vi "getProcessName.vi"(10 "Lotno":string) -> (2 "ProcessName":string)   [LabVIEW 2012]
uses:
  <vilib>/addons/database/Auxilliary.llb/DB Tools Cursor Type.ctl
  <vilib>/addons/database/Connection.llb/DB Tools Open Connec (Path).vi
  <vilib>/addons/database/Connection.llb/Conn Execute.vi
  <vilib>/addons/database/Recordset.llb/Rec Fetch Integer Data (R).vi
  <vilib>/addons/database/Recordset.llb/Rec Destroy - Connection.vi
  <vilib>/addons/database/Recordset.llb/Rec Fetch Recordset Data (R).vi
  <vilib>/addons/database/_DB Variant To Data/Database Variant To Data.xnode
  <vilib>/addons/database/NI_Database_API.lvlib
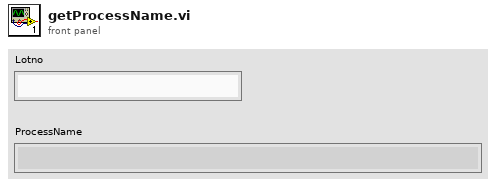
[diagram p1: front panel]
types:
  T1 = typedef "NI_Database_API.lvlib/DB Tools Cursor Type.ctl" = enum16{"forward-only", "keyset", "dynamic", "static"}
  T2 = typedef "NI_Database_API.lvlib/Conn ObjectReference.ctl" = refnum<k1>
  T3 = typedef "NI_Database_API.lvlib/Rec ObjectReference.ctl" = refnum<k1>
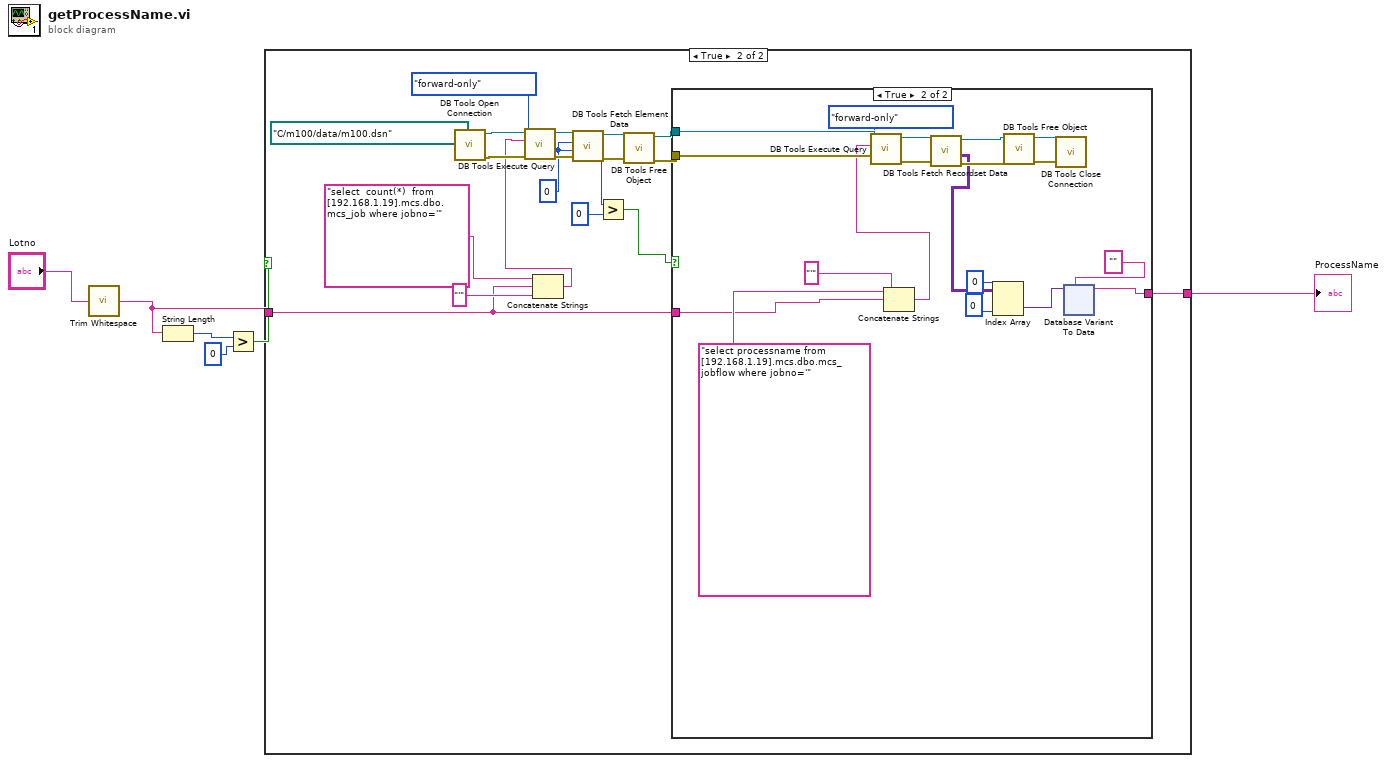
[diagram p0: block diagram]
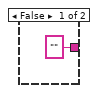
[diagram p2: hidden frame]
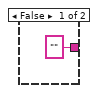
[diagram p3: hidden frame]
diagram:
  n1 = call <vilib>:"Trim Whitespace.vi"("string"="Lotno") -> ("trimmed string"=w2:string)  [unwired: 1 in]
  n2 = String Length(string=w2) -> (length=w6:i32)
  n3 = Greater?(x=w6, y=0) -> (0:w4:bool)
  n4 = case shown="True" w4 {
    tunnel: w2 -> [_ w19]
    tunnel: ["" ("data") w26] -> w1
    frame False {
    }
    frame True {
      w12 = 0
      n5 = call-poly <vilib>:"DB Tools Open Connection.vi"("connection information"=path "C:/m100/data/m100.dsn") -> ("error out"=w22:errorcluster, "connection reference"=w23:T2)  [unwired: 7 in]
      n6 = Concatenate Strings("select  count(*)  from [192.168.1.19].mcs.dbo.mcs_job where jobno='" ("string"), w19, "'" ("string")) -> (w17:string)
      n7 = call-poly <vilib>:"DB Tools Execute Query.vi"("error in (no error)"=w22, "cursor type"=DB_Tools_Cursor_Type."forward-only", "SQL query"=w17, "connection reference"=w23) -> ("error out"=w16:errorcluster, "recordset reference"=w15:T3)  [unwired: 4 in]
      n8 = call-poly <vilib>:"DB Tools Fetch Element Data.vi"("error in (no error)"=w16, "type"=w12, "column index"=w12, "recordset reference"=w15) -> ("error out"=w13:errorcluster, "data"=w11:i32, "recordset reference out"=w14:T3)  [unwired: 3 in]
      n9 = Greater?(x=w11, y=0) -> (0:w9:bool)
      n10 = call-poly <vilib>:"DB Tools Free Object.vi"("error in (no error)"=w13, "recordset reference"=w14) -> ("error out"=w24:errorcluster, "connection reference"=w25:T2)  [unwired: 8 in]
      n11 = case shown="True" w9 {
        tunnel: w25 -> [_ w44]
        tunnel: w24 -> [_ w41]
        tunnel: w19 -> [_ w32]
        tunnel: ["" ("data") w31] -> w26
        frame False {
        }
        frame True {
          n12 = Concatenate Strings("select processname from [192.168.1.19].mcs.dbo.mcs_jobflow where jobno='" ("string"), w32, "'" ("string")) -> (w35:string)
          n13 = call-poly <vilib>:"DB Tools Execute Query.vi"("error in (no error)"=w41, "cursor type"=DB_Tools_Cursor_Type."forward-only", "SQL query"=w35, "connection reference"=w44) -> ("error out"=w40:errorcluster, "recordset reference"=w43:T3)  [unwired: 4 in]
          n14 = call-poly <vilib>:"DB Tools Fetch Recordset Data.vi"("error in (no error)"=w40, "recordset reference"=w43) -> ("error out"=w39:errorcluster, "recordset data"=w30:variant[][], "recordset reference out"=w42:T3)  [unwired: 3 in]
          n15 = Index Array(array=w30, index (row)=0 ("disabled index (row)"), index (col)=0 ("disabled index (col)")) -> (element=w33:variant)
          n16 = call-poly <vilib>:"DB Tools Free Object.vi"("error in (no error)"=w39, "recordset reference"=w42) -> ("error out"=w46:errorcluster, "connection reference"=w45:T2)  [unwired: 8 in]
          n17 = call <vilib>:"DB Tools Close Connection.vi"("error in (no error)"=w46, "connection reference"=w45) -> ()  [unwired: 5 in, 1 out]
          n18 = xnode "Database Variant To Data"("database variant"=w33, "type"="") -> ("data"=w31:string)  [unwired: 1 in, 1 out]
        }
      }
    }
  }
  "ProcessName" <- w1
